vi "SPC_close_phot_stream.vi"(6 "Stream Handle":i16, 8 "Error In":errorcluster, 11 "DLL Path":path) -> (0 "Error Out":errorcluster, 3 "DLL Path":path, 4 "Stream Handle":i16)   [LabVIEW 2017]
doc: "The procedure is used to close the opened photons stream defined by handle 'stream_hndl' after extraction of the photons.\nThe procedure frees all stream's memory and finally invalidates the handle 'stream_hndl'. \nProcedure returns error, if 'stream_hndl' is not the handle of the stream opened using \nSPC_init_phot_stream function.\n\ninfo@becker-hickl.com"
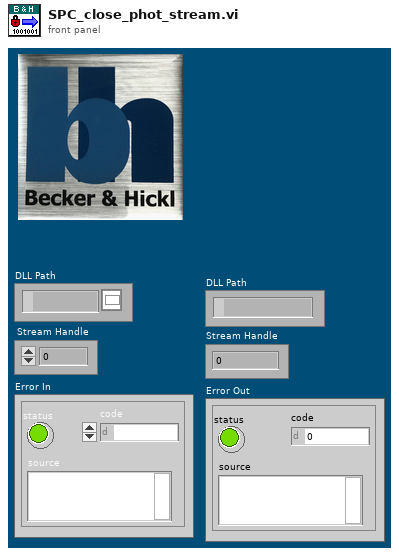
[diagram p1: front panel]
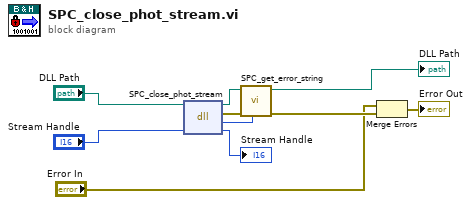
[diagram p0: block diagram]
diagram:
  n1 = dll-call lib="D:/spcm/lib/lab_view/lv10.0/spcm32.dll" fn="SPC_close_phot_stream"(path in="DLL Path", "stream_hndl"="Stream Handle") -> (path out=w4:path, error out=w5:errorcluster, "return type"=w3:i16, "stream_hndl"=→"Stream Handle":i16)  [unwired: 2 in]
  n2 = call "SPC_get_error_string.vi"("ErrorID"=w3, "Error In"=w5, "DLL Path"=w4) -> ("Error Out"=w8:errorcluster, "DLL Path"=→"DLL Path":path)  [unwired: 6 in, 1 out]
  n3 = Merge Errors("Error In", w8) -> (→"Error Out":errorcluster)
